vi "Encrypt.vi"(1 "String":string) -> (0 "Encrypted String":string)   [LabVIEW 2016, in "UserPwd DB.lvlib" / "UserPwd DB.lvclass"]
uses:
  <userlib>/Common Components/UserPwd DB/UserPwd DB/UserPwd DB.lvclass
  <userlib>/_OpenG.lib/md5/md5.llb/MD5 Message Digest (Hexadecimal String)__ogtk.vi
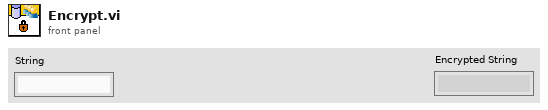
[diagram p1: front panel]
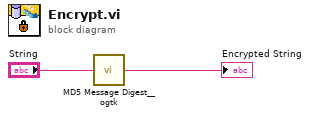
[diagram p0: block diagram]
diagram:
  n1 = call-poly <userlib>:"MD5 Message Digest__ogtk.vi"("Message"="String") -> ("MD5 Message Digest"=→"Encrypted String":string)
